vi "Draw_Build Region bounds and Position.vi"(0 "Postion":T1, 1 "Height":u32, 2 "Width":u32, 3 "Error In":errorcluster) -> (7 "Region Out":T2, 10 "Error Out":errorcluster)   [LabVIEW 2009]
uses:
  Controls/Cluster/Cluster_Region info.ctl
  Controls/Cluster/Cluster_Top Left position.ctl
panel:
  # "Copyright (C) 2005 Mark Balla mballa@sbcglobal.net\n\nThis library is free software; you can redistribute it and/or\nmodify it.\n\nThis library is distributed in the hope that it will be useful,\nbut WITHOUT ANY WARRANTY; without even the implied warranty of\nMERCHANTABILITY or FITNESS FOR A PARTICULAR PURPOSE."
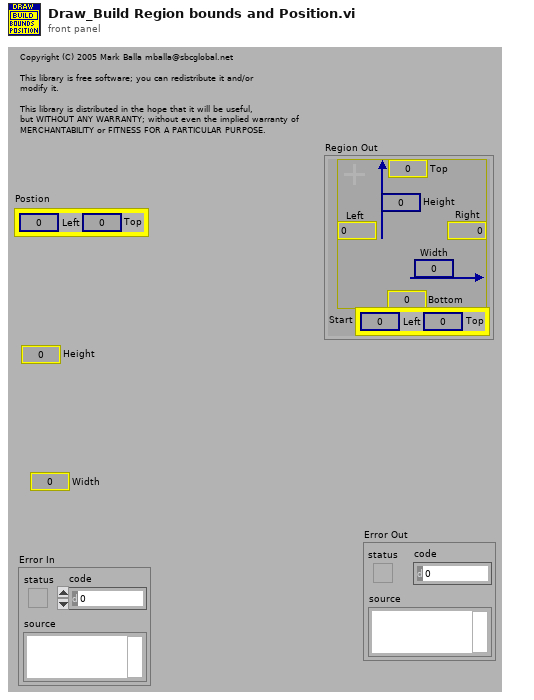
[diagram p1: front panel]
types:
  T1 = typedef "Cluster_Top Left position.ctl" = cluster{"Left":i32, "Top":i32}
  T2 = typedef "Cluster_Region info.ctl" = cluster{"Left":i32, "Top":i32, "Right":i32, "Bottom":i32, "Width":u32, "Height":u32, "Start":T1}
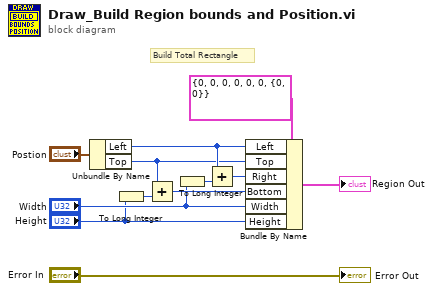
[diagram p0: block diagram]
diagram:
  # "Build Total Rectangle"
  n1 = Unbundle By Name("Postion") -> ("Left"=w7:i32, "Top"=w6:i32)
  n2 = To Long Integer(number="Height") -> (32bit integer=w1:i32)
  n3 = Add(x=w6, y=w1) -> (x+y=w5:i32)
  n4 = To Long Integer(number="Width") -> (32bit integer=w4:i32)
  n5 = Add(x=w7, y=w4) -> (x+y=w8:i32)
  n6 = Bundle By Name(cluster=T2 {"Left"=0, "Top"=0, "Right"=0, "Bottom"=0, "Width"=0, "Height"=0, "Start"={"Left"=0, "Top"=0}} ("Rectangle Out"), "Left"=w7, "Top"=w6, "Right"=w8, "Bottom"=w5, "Width"="Width", "Height"="Height") -> (→"Region Out":T2)
  "Error Out" <- "Error In"
